vi "startValueChange.vi"(8 "error in (no error)":errorcluster, 9 "oldValue":dbl, 10 "newValue":dbl, 11 "ScanCreator in":refnum<class "ScanCreator.lvclass">) -> (0 "error out":errorcluster, 3 "ScanCreator out":refnum<class "ScanCreator.lvclass">)   [LabVIEW 2009, in "Views.lvlib" / "ScriptEditor.lvlib" / "ScanCreator.lvclass"]
uses:
  ScanCreator.lvclass
  ScanCreator.lvclass/ScanCreator.ctl
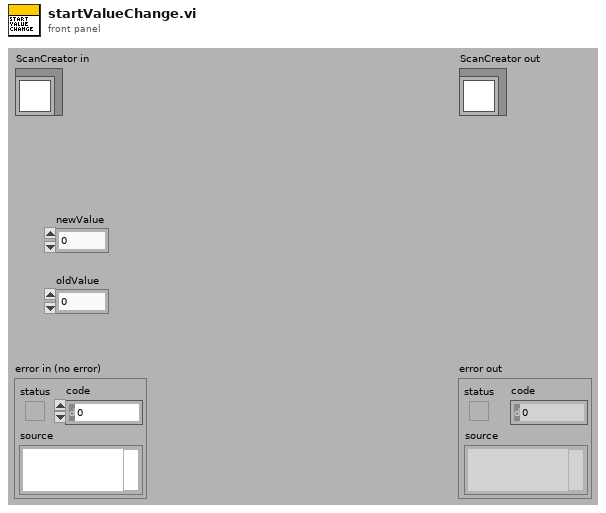
[diagram p1: front panel]
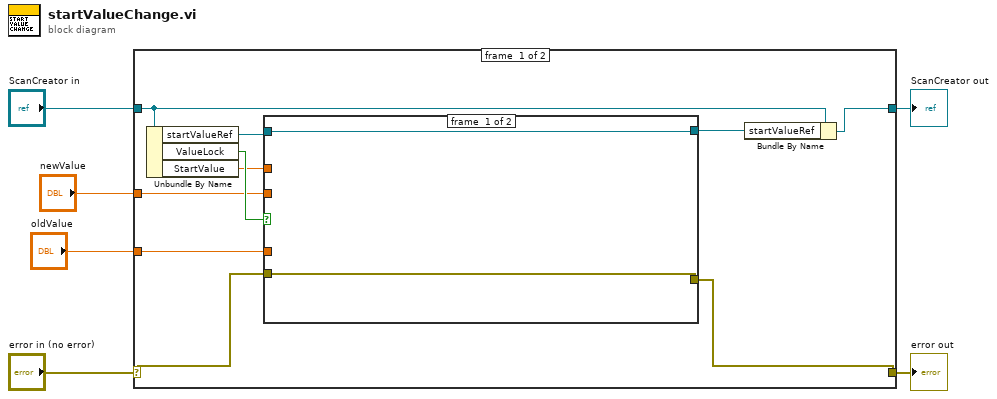
[diagram p0: block diagram]
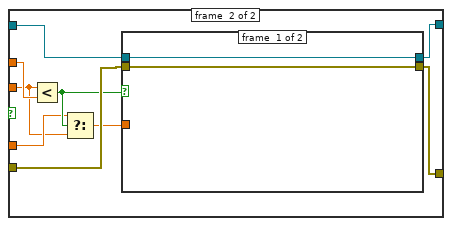
[diagram p2: hidden frame]
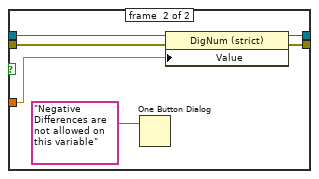
[diagram p3: hidden frame]
diagram:
  n1 = case shown="No Error" "error in (no error)" {
    selector: "error in (no error)" -> [w11 w37]
    tunnel: [w10 w37] -> w5
    tunnel: [w8 w36] -> w3
    tunnel: "ScanCreator in" -> [w9 w36]
    tunnel: "newValue" -> [w14 _]
    tunnel: "oldValue" -> [w13 _]
    frame #0 {
      n2 = Unbundle By Name(w9) -> ("startValueRef"=w12:refnum<vi>, "ValueLock"=w16:bool, "StartValue"=w15:dbl)
      n3 = case shown="True" w16 {
        tunnel: w15 -> [_ w27]
        tunnel: w14 -> [_ w21]
        tunnel: w13 -> [_ w22]
        tunnel: w12 -> [w18 w26]
        tunnel: w11 -> [w17 w25]
        tunnel: [w17 w24] -> w10
        tunnel: [w18 w19] -> w7
        frame #0 {
        }
        frame #1 {
          n4 = Less?(x=w21, y=w27) -> (x < y?=w23:bool)
          n5 = Select(t=w22, s=w23, f=w21) -> (s? t:f=w20:dbl)
          n6 = case shown="True" w23 {
            tunnel: w26 -> [w29 w34]
            tunnel: w25 -> [w28 w33]
            tunnel: [w28 w32] -> w24
            tunnel: w20 -> [_ w31]
            tunnel: [w29 w30] -> w19
            frame #0 {
            }
            frame #1 {
              n7 = One Button Dialog(message="Negative Differences are not allowed on this variable") -> ()  [unwired: 1 in, 1 out]
              n8 = property class="DigNum (strict)"(reference=w34, error in=w33, "Value"=w31) -> (reference out=w30:refnum<vi>, error out=w32:errorcluster)
            }
          }
        }
      }
      n9 = Bundle By Name(cluster=w9, "startValueRef"=w7) -> (w8:refnum<class "ScanCreator.lvclass">)
    }
    frame #1 {
    }
  }
  "error out" <- w5
  "ScanCreator out" <- w3
